vi "Get_Handle.vi"(9 "password":string="gamma2018", 11 "username":string="admin") -> (3 "Refnum out":T1)   [LabVIEW 2016]
uses:
  <vilib>/httpClient/ClientHandle.ctl
  <vilib>/httpClient/LabVIEWHTTPClient.lvlib
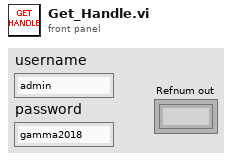
[diagram p1: front panel]
types:
  T1 = typedef "LabVIEWHTTPClient.lvlib/ClientHandle.ctl" = refnum<k1>
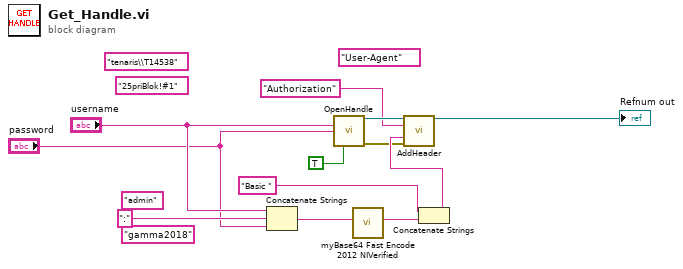
[diagram p0: block diagram]
diagram:
  (unwired) "25priBlok!#1" ("password")
  (unwired) "tenaris\\T14538" ("username")
  (unwired) "gamma2018"
  (unwired) "admin"
  (unwired) "User-Agent" ("header")
  n1 = Concatenate Strings("username", ":", "password") -> (w4:string)
  n2 = call <vilib>:"OpenHandle.vi"("username"="username", "password"="password", "verify server(true)"=TRUE) -> ("client handle out"=w11:T1, "error out"=w6:errorcluster)  [unwired: 11 in]
  n3 = call "myBase64 Fast Encode 2012 NIVerified.vi"("string in (not encoded)"=w4) -> ("string out (base64-encoded)"=w10:string)  [unwired: 9 in, 1 out]
  n4 = Concatenate Strings("Basic ", w10) -> (w8:string)
  n5 = call <vilib>:"AddHeader.vi"("client handle"=w11, "header"="Authorization", "value"=w8, "error in (no error)"=w6) -> ("client handle out"=→"Refnum out":T1)  [unwired: 10 in, 1 out]
